vi "Debug.vi"(11 "SOL-Config in":refnum<class "SOL-Config.lvclass">) -> (2 "Debug":bool, 3 "SOL-Config out":refnum<class "SOL-Config.lvclass">)   [LabVIEW 2020, in "Summer of LabVIEW.lvlib" / "SOL-Config.lvclass"]
uses:
  SOL-Config.lvclass
  SOL-Config.lvclass/SOL-Config.ctl
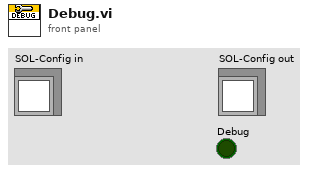
[diagram p1: front panel]
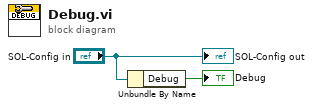
[diagram p0: block diagram]
diagram:
  n1 = Unbundle By Name("SOL-Config in") -> ("Debug"=→"Debug":bool)
  "SOL-Config out" <- "SOL-Config in"
